vi "VehiclePosition_Interface.vi"(8 "error in":errorcluster) -> (0 "error out":errorcluster)   [LabVIEW 2019]
uses:
  #typedef_Queue_enum.ctl
  #typedef_VehiclePosition_Action_enum.ctl
  #typedef_Data_VehiclePos.ctl
  #typedef_Data_Controller.ctl
  #typedef_EntryConsole_Action_enum.ctl
  #typedef_WashDisplay_Action_enum.ctl
  #typedef_Controller_Action_enum.ctl
  #typedef_VehiclePos_enum.ctl
  #typedef_WashStepInfo.ctl
  #typedef_WashStates.ctl
panel:
  in  "Vehicle Position Simulation":u8(slide) caption="Slide" scale=0.0..4.0
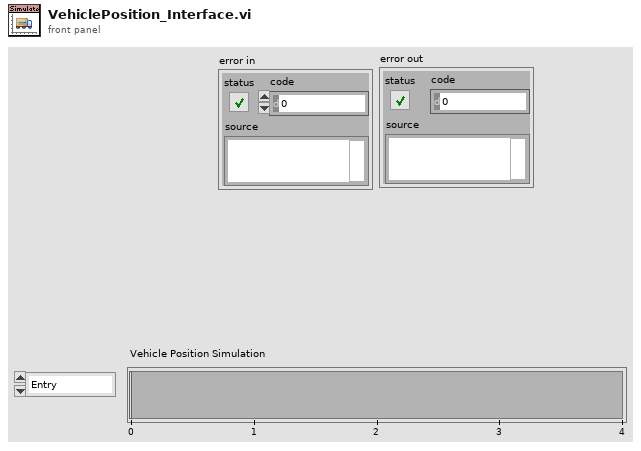
[diagram p1: front panel]
types:
  T1 = typedef "#typedef_Queue_enum.ctl" = enum16{"ERROR_default", "Obtain", "Enqueue", "GetStatus", "Flush", "Release"}
  T2 = typedef "#typedef_Data_VehiclePos.ctl" = cluster{"VehiclePosSimulation":i8, "VehiclePosition_Action":T3}
  T3 = typedef "#typedef_VehiclePosition_Action_enum.ctl" = enum16{"Init", "ERROR_DEFAULT", "Idle", "Close", "Error_Handler", "Exit", "Send Vehicle Pos"}
  T4 = typedef "#typedef_Data_Controller.ctl" = cluster{"EntryConsole_Action":T5, "WashDisplay_Action":T6, "Controller_Action":T7, "VehiclePosition_Action":T3, "Under Body Wash":bool, "Bug Remover":bool, "Pre-Soak":bool, "High Pressure Wash (default)":bool, "Low Pressure Wax":bool, "Spot Free Rinse":bool, "Tire Shine Foam":bool, "Air Dry":bool, "Start":bool, "Current Vehicle Pos":T8, "Steps List":T9[], "Current Step Ind":i32}
  T5 = typedef "#typedef_EntryConsole_Action_enum.ctl" = enum16{"Init", "ERROR_DEFAULT", "Idle", "Start_Wash_Cycle", "Clear_Console", "Close", "Error_Handler", "Exit"}
  T6 = typedef "#typedef_WashDisplay_Action_enum.ctl" = enum16{"Init", "ERROR_DEFAULT", "Idle", "Update FP", "Close", "Error_Handler", "Exit"}
  T7 = typedef "#typedef_Controller_Action_enum.ctl" = enum16{"ERROR_DEFAULT", "Init", "Read database", "(Idle) Wait for Start", "Start", "Wait for Vehicle Pos", "Wash Step Execution", "Wash Completion", "Wash Exit", "Wash Abort", "Close", "Error Handler", "Exit"}
  T8 = typedef "#typedef_VehiclePos_enum.ctl" = u8
  T9 = typedef "#typedef_WashStepInfo.ctl" = cluster{"Wash States":T10, "Expected Vehicle Pos":i32, "Step duration":i32}
  T10 = typedef "#typedef_WashStates.ctl" = enum16{"Under Body Wash", "Bug Remover", "Pre-Soak", "High Pressure Wash", "Low Pressure Wax", "Spot Free Rinse", "Tire Shine Foam", "Air Dry"}
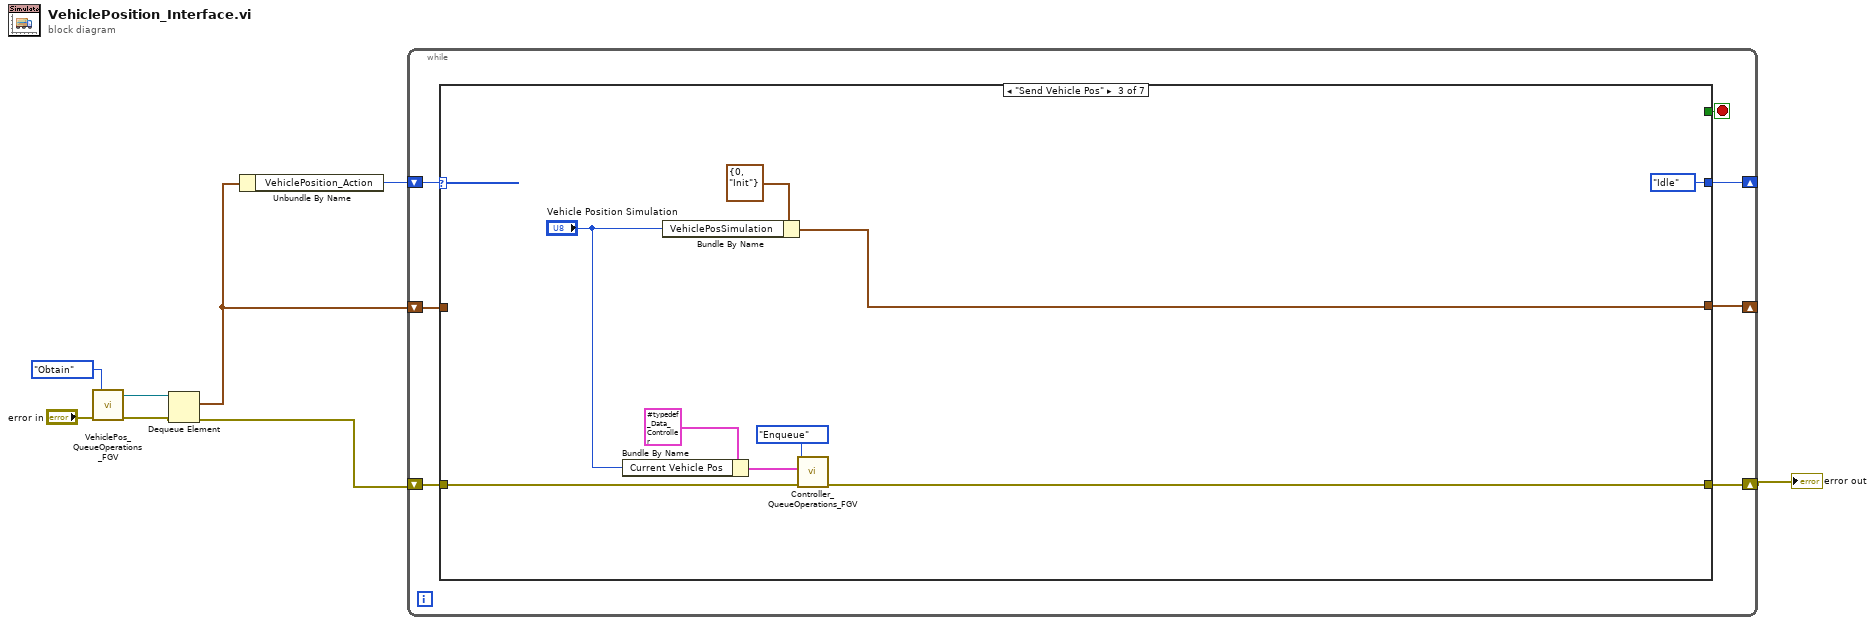
[diagram p0: block diagram]
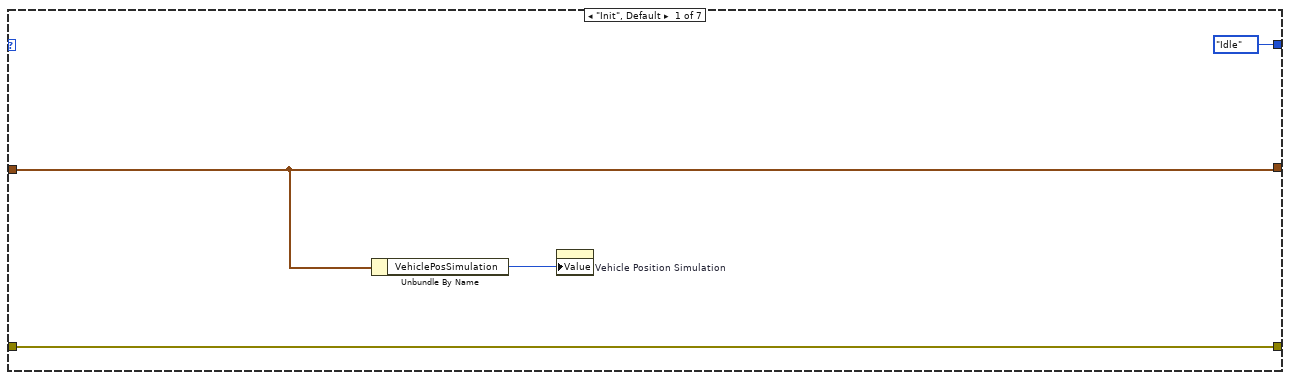
[diagram p2: hidden frame]
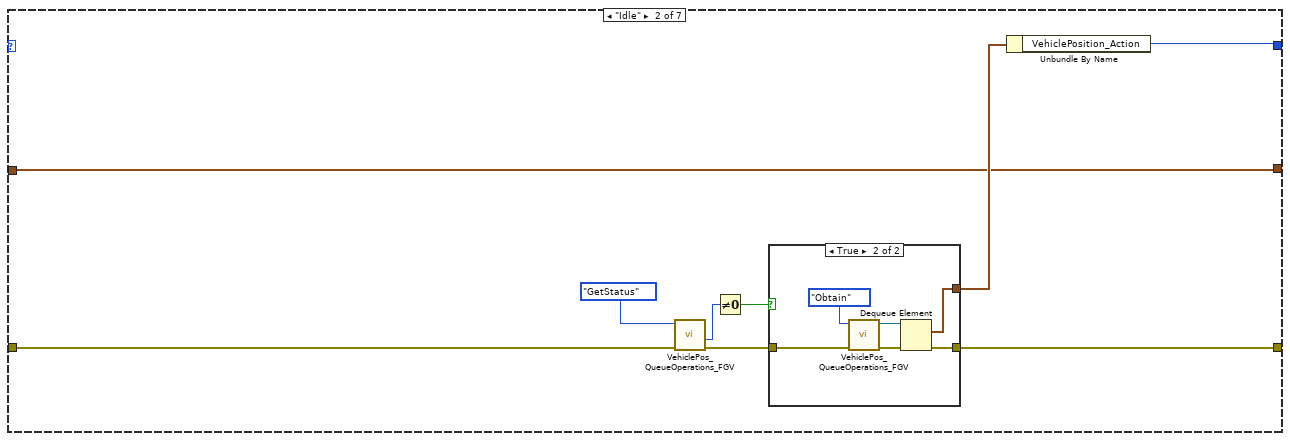
[diagram p3: hidden frame]
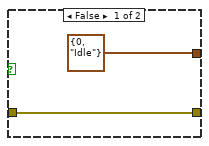
[diagram p4: hidden frame]
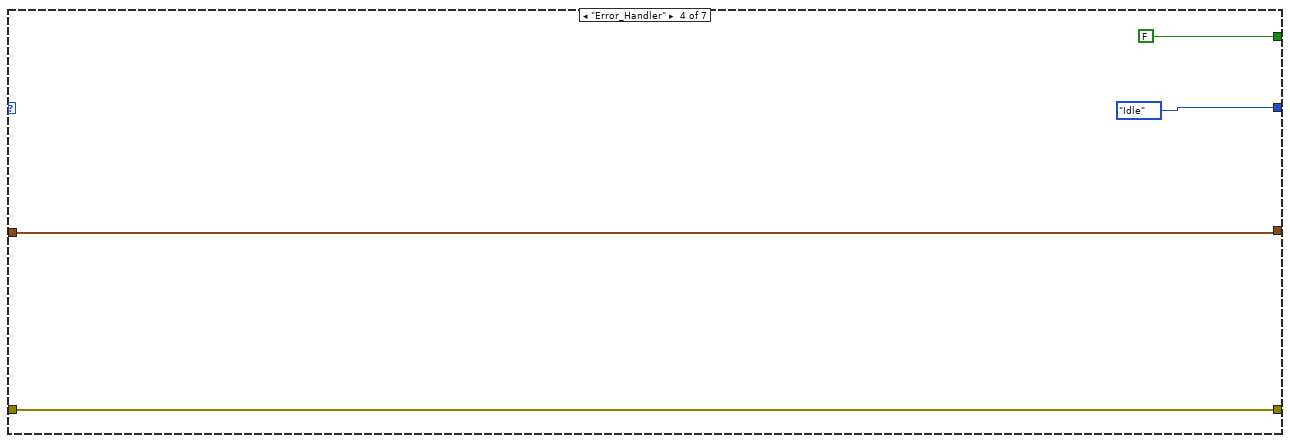
[diagram p5: hidden frame]
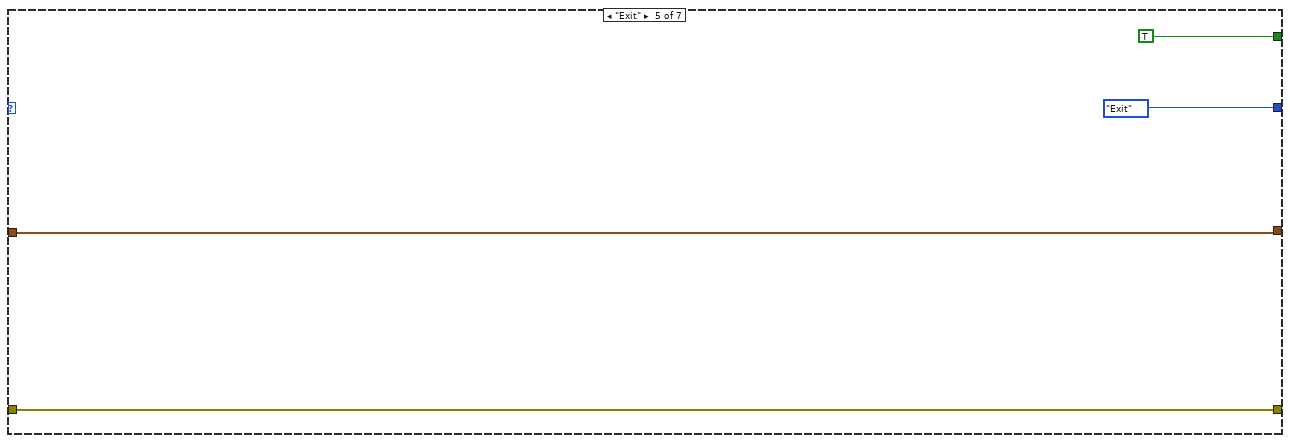
[diagram p6: hidden frame]
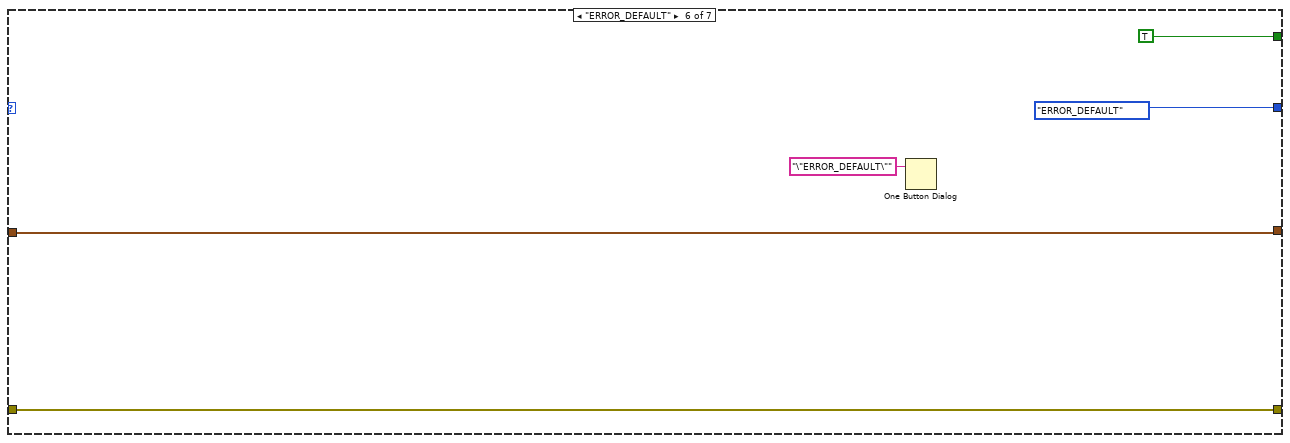
[diagram p7: hidden frame]
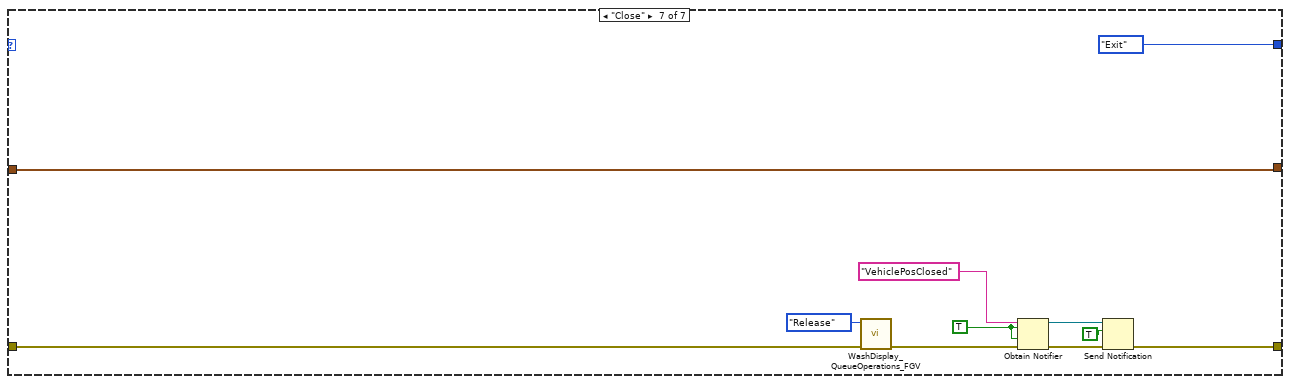
[diagram p8: hidden frame]
diagram:
  n1 = call "VehiclePos_QueueOperations_FGV.vi"("error in"="error in", "Action"=#typedef_Queue_enum."Obtain") -> ("error out"=w6:errorcluster, "queue ref"=w7:refnum<queue>)  [unwired: 6 in, 2 out]
  n2 = Dequeue Element(queue=w7, error in (no error)=w6) -> (element=w3:T2, error out=w4:errorcluster)  [unwired: 1 in, 2 out]
  n3 = Unbundle By Name(w3) -> ("VehiclePosition_Action"=w2:T3)
  n4 = while {
    shift-right: [w14] -> _
    shift-left: w2 -> [w15]
    shift-right: [w12] -> _
    shift-left: w3 -> [w9]
    shift-right: [w10] -> w1
    shift-left: w4 -> [w11]
    stop <- w13 stop-if-true
    n5 = case shown="\"Send Vehicle Pos\"" w15 {
      tunnel: [#typedef_VehiclePosition_Action_enum."Idle" ("VehiclePosition_Action") w22 #typedef_VehiclePosition_Action_enum."Idle" ("VehiclePosition_Action") #typedef_VehiclePosition_Action_enum."Idle" ("VehiclePosition_Action") #typedef_VehiclePosition_Action_enum."Exit" ("VehiclePosition_Action") #typedef_VehiclePosition_Action_enum."ERROR_DEFAULT" ("VehiclePosition_Action") #typedef_VehiclePosition_Action_enum."Exit" ("VehiclePosition_Action")] -> w14
      tunnel: [_ _ _ FALSE TRUE TRUE _] -> w13
      tunnel: [w17 w20 w43 w46 w50 w54 w59] -> w12
      tunnel: w11 -> [w19 w23 w44 w48 w52 w56 w69]
      tunnel: [w19 w21 w45 w48 w52 w56 w63] -> w10
      tunnel: w9 -> [w17 w20 _ w46 w50 w54 w59]
      frame "Init", Default {
        n6 = Unbundle By Name(w17) -> ("VehiclePosSimulation"=w16:i8)
        n7 = property on="Vehicle Position Simulation" class="Slide (strict)"("Value"=w16) -> ()  [unwired: 2 in, 2 out]
      }
      frame "Idle" {
        n8 = call "VehiclePos_QueueOperations_FGV.vi"("error in"=w23, "Action"=#typedef_Queue_enum."GetStatus") -> ("error out"=w27:errorcluster, "#elements in queue"=w26:i32)  [unwired: 6 in, 2 out]
        n9 = Not Equal To 0?(x=w26) -> (x != 0?=w25:bool)
        n10 = case shown="True" w25 {
          tunnel: w27 -> [w30 w35]
          tunnel: [w30 w33] -> w21
          tunnel: [T2 {"VehiclePosSimulation"=0, "VehiclePosition_Action"=enum."Idle"} ("Data") w31] -> w28
          frame False {
          }
          frame True {
            n11 = call "VehiclePos_QueueOperations_FGV.vi"("error in"=w35, "Action"=#typedef_Queue_enum."Obtain") -> ("error out"=w34:errorcluster, "queue ref"=w32:refnum<queue>)  [unwired: 6 in, 2 out]
            n12 = Dequeue Element(queue=w32, error in (no error)=w34) -> (element=w31:T2, error out=w33:errorcluster)  [unwired: 1 in, 2 out]
          }
        }
        n13 = Unbundle By Name(w28) -> ("VehiclePosition_Action"=w22:T3)
      }
      frame "Send Vehicle Pos" {
        n14 = Bundle By Name(cluster=T4 {"EntryConsole_Action"=enum."Init", "WashDisplay_Action"=enum."Init", "Controller_Action"=enum."Init", "VehiclePosition_Action"=enum."Init", "Under Body Wash"=FALSE, "Bug Remover"=FALSE, "Pre-Soak"=FALSE, "High Pressure Wash (default)"=FALSE, "Low Pressure Wax"=FALSE, "Spot Free Rinse"=FALSE, "Tire Shine Foam"=FALSE, "Air Dry"=FALSE, "Start"=FALSE, "Current Vehicle Pos"=1, "Steps List"=[], "Current Step Ind"=0} ("Data"), "Current Vehicle Pos"="Vehicle Position Simulation") -> (w41:T4)
        n15 = Bundle By Name(cluster=T2 {"VehiclePosSimulation"=0, "VehiclePosition_Action"=enum."Init"} ("Data"), "VehiclePosSimulation"="Vehicle Position Simulation") -> (w43:T2)
        n16 = call "Controller_QueueOperations_FGV.vi"("error in"=w44, "Data In"=w41, "Action"=#typedef_Queue_enum."Enqueue") -> ("error out"=w45:errorcluster)  [unwired: 5 in, 3 out]
      }
      frame "Error_Handler" {
      }
      frame "Exit" {
      }
      frame "ERROR_DEFAULT" {
        n17 = One Button Dialog(message="\"ERROR_DEFAULT\"") -> ()  [unwired: 1 in, 1 out]
      }
      frame "Close" {
        w61 = TRUE
        n18 = call "WashDisplay_QueueOperations_FGV.vi"("error in"=w69, "Action"=#typedef_Queue_enum."Release") -> ("error out"=w67:errorcluster)  [unwired: 6 in, 3 out]
        n19 = Obtain Notifier(name (unnamed)="VehiclePosClosed", notification data type=w61, create if not found? (T)=w61, error in (no error)=w67) -> (notifier out=w62:refnum<notifier>, error out=w64:errorcluster)  [unwired: 1 out]
        n20 = Send Notification(notification=TRUE, notifier=w62, error in (no error)=w64) -> (error out=w63:errorcluster)  [unwired: 1 out]
      }
    }
  }
  "error out" <- w1
